vi "test-matrix.vi"(8 "error in (no error)":errorcluster) -> (0 "error out":errorcluster, 3 "All Tests\nPassed":bool)   [LabVIEW 2019]
uses:
  <vilib>/Analysis/baseanly.llb/Real A x B.vi
  <vilib>/Rock Robotics/WPI/ThirdParty/JAS_Junk/TrajLib/MatBuilder_Create.vi
  <vilib>/Analysis/7linalg.llb/Matrix Exp.vi
  <vilib>/Analysis/7linalg.llb/Real Matrix Exp.vi
  <vilib>/Analysis/7linalg.llb/Solve Linear Equations (multiple right hand).vi
  <vilib>/Analysis/baseanly.llb/Real Inverse Matrix.vi
  <vilib>/Analysis/7linalg.llb/Create Special Matrix.vi
  <vilib>/Analysis/7linalg.llb/Create Special Real Matrix.vi
  <vilib>/Analysis/Matrix/Numeric/Add/Add (Elementwise) - RM,R.vi
  <vilib>/Analysis/Matrix/Numeric/Multiply/Multiply - RM,R.vi
  <vilib>/Analysis/Matrix/Numeric/Subtract/Subtract (Elementwise) - RM,R.vi
  <vilib>/Analysis/Matrix/Numeric/Add/Add - RM,RM.vi
  <vilib>/Analysis/Matrix/Numeric/Subtract/Subtract - RM,RM.vi
  <vilib>/Rock Robotics/WPI/ThirdParty/JAS_Junk/TrajLib/Trajectory_Library.lvlib
  <vilib>/Analysis/NI_AALBase.lvlib
  <vilib>/Analysis/NI_AALPro.lvlib
  <vilib>/Analysis/Matrix/NI_Matrix.lvlib
panel:
  out "Test Passed 8-1":bool
  out "Test Passed 8-0":bool
  out "Test Passed 7-1":bool
  out "Test Passed 7-0":bool
  out "Test Passed 6-3":bool
  out "Test Passed 6-2":bool
  out "Test Passed 6-1":bool
  out "Test Passed 6-0":bool
  out "Test Passed 5-0":bool
  out "Test Passed 4-0":bool
  out "Test Passed 3-1":bool
  out "Test Passed 3-0":bool
  out "Test Passed 2-0":bool
  out "Test Passed 1-0":bool
  out "Test Passed 0-1":bool
  out "Test Passed 0-0":bool
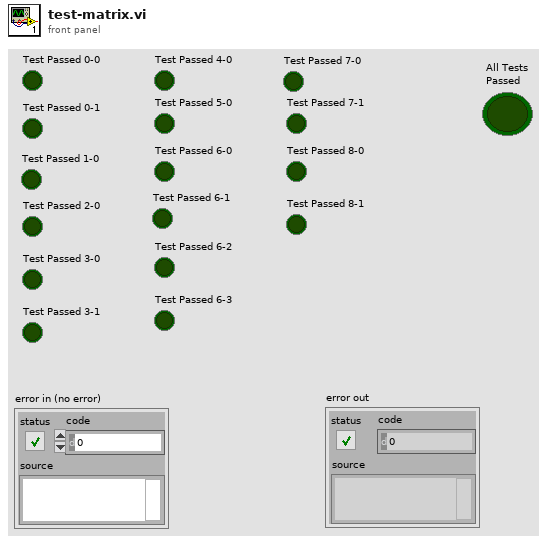
[diagram p1: front panel]
types:
  T1 = typedef "NI_Matrix.lvlib/RealMatrix.ctl" = dbl[][]
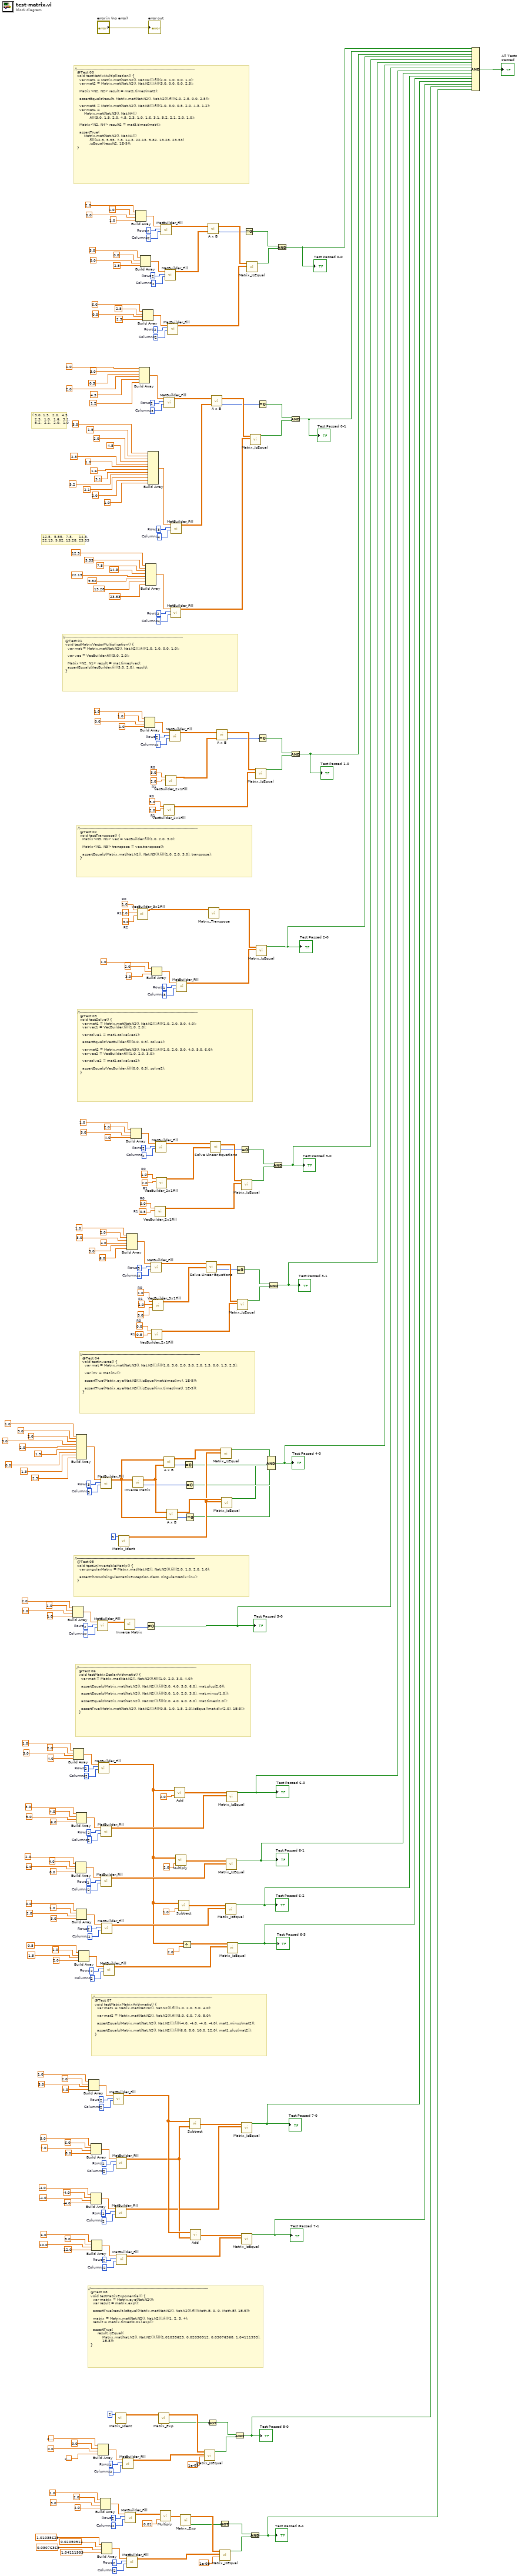
[diagram p0: block diagram]
diagram:
  w13 = 2  # Columns
  w12 = 2  # Rows
  w32 = 2  # Columns
  w31 = 2  # Rows
  w39 = 2  # Columns
  w38 = 2  # Rows
  w50 = 2  # Columns
  w49 = 2  # Rows
  w57 = 2  # Columns
  w56 = 2  # Rows
  w64 = 2  # Columns
  w63 = 2  # Rows
  w71 = 2  # Columns
  w70 = 2  # Rows
  w95 = 2  # Columns
  w94 = 2  # Rows
  w102 = 2  # Columns
  w101 = 2  # Rows
  w109 = 2  # Columns
  w108 = 2  # Rows
  w116 = 2  # Columns
  w115 = 2  # Rows
  w123 = 2  # Columns
  w122 = 2  # Rows
  w133 = 2  # Columns
  w132 = 2  # Rows
  w162 = 3  # Columns
  w161 = 3  # Rows
  w179 = 0.5  # R1
  w178 = 0.0  # R0
  w181 = 2.0  # R1
  w180 = 1.0  # R0
  w183 = 2  # Columns
  w182 = 3  # Rows
  w209 = 0.5  # R1
  w208 = 0.0  # R0
  w211 = 2.0  # R1
  w210 = 1.0  # R0
  w213 = 2  # Columns
  w212 = 2  # Rows
  w225 = 3.0  # R2
  w224 = 2.0  # R1
  w223 = 1.0  # R0
  w227 = 3  # Columns
  w226 = 1  # Rows
  w234 = 2.0  # R1
  w233 = 5.0  # R0
  w237 = 2.0  # R1
  w236 = 3.0  # R0
  w241 = 2  # Columns
  w240 = 2  # Rows
  w265 = 4  # Columns
  w264 = 2  # Rows
  w274 = 4  # Columns
  w273 = 3  # Rows
  w281 = 3  # Columns
  w280 = 2  # Rows
  w290 = 2  # Columns
  w289 = 2  # Rows
  w299 = 2  # Columns
  w298 = 2  # Rows
  w306 = 2  # Columns
  w305 = 2  # Rows
  # "//----------------------------------------------------------------------------------------------------\n  @Test 07\n  void testMatrixMatrixArithmetic() {\n    var mat1 = Matrix.mat(Nat.N2(), Nat.N2()).fill(1.0, 2.0, 3.0, 4.0);\n\n    var mat2 = Matrix.mat(Nat.N2(), Nat.N2()).fill(5.0, 6.0, 7.0, 8.0);\n\n    assertEquals(Matrix.mat(Nat.N2(), Nat.N2()).fill(-4.0, -4.0, -4.0, -4.0), mat1.minus(mat2));\n\n    assertEquals(Matrix.mat(Nat.N2(), Nat.N2()).fill(6.0, 8.0, 10.0, 12.0), mat1.plus(mat2));\n  }"
  # "//----------------------------------------------------------------------------------------------------\n  @Test 06\n  void testMatrixScalarArithmetic() {\n    var mat = Matrix.mat(Nat.N2(), Nat.N2()).fill(1.0, 2.0, 3.0, 4.0);\n\n    assertEquals(Matrix.mat(Nat.N2(), Nat.N2()).fill(3.0, 4.0, 5.0, 6.0), mat.plus(2.0));\n\n    assertEquals(Matrix.mat(Nat.N2(), Nat.N2()).fill(0.0, 1.0, 2.0, 3.0), mat.minus(1.0));\n\n    assertEquals(Matrix.mat(Nat.N2(), Nat.N2()).fill(2.0, 4.0, 6.0, 8.0), mat.times(2.0));\n\n    assertTrue(Matrix.mat(Nat.N2(), Nat.N2()).fill(0.5, 1.0, 1.5, 2.0).isEqual(mat.div(2.0), 1E-3));\n  }"
  # "//----------------------------------------------------------------------------------------------------\n  @Test 05\n  void testUninvertableMatrix() {\n    var singularMatrix = Matrix.mat(Nat.N2(), Nat.N2()).fill(2.0, 1.0, 2.0, 1.0);\n\n    assertThrows(SingularMatrixException.class, singularMatrix::inv);\n  }"
  # "//----------------------------------------------------------------------------------------------------\n  @Test 04\n  void testInverse() {\n    var mat = Matrix.mat(Nat.N3(), Nat.N3()).fill(1.0, 3.0, 2.0, 5.0, 2.0, 1.5, 0.0, 1.3, 2.5);\n\n    var inv = mat.inv();\n\n    assertTrue(Matrix.eye(Nat.N3()).isEqual(mat.times(inv), 1E-9));\n\n    assertTrue(Matrix.eye(Nat.N3()).isEqual(inv.times(mat), 1E-9));\n  }"
  # "//----------------------------------------------------------------------------------------------------\n  @Test 03\n  void testSolve() {\n    var mat1 = Matrix.mat(Nat.N2(), Nat.N2()).fill(1.0, 2.0, 3.0, 4.0);\n    var vec1 = VecBuilder.fill(1.0, 2.0);\n\n    var solve1 = mat1.solve(vec1);\n\n    assertEquals(VecBuilder.fill(0.0, 0.5), solve1);\n\n    var mat2 = Matrix.mat(Nat.N3(), Nat.N2()).fill(1.0, 2.0, 3.0, 4.0, 5.0, 6.0);\n    var vec2 = VecBuilder.fill(1.0, 2.0, 3.0);\n\n    var solve2 = mat2.solve(vec2);\n\n    assertEquals(VecBuilder.fill(0.0, 0.5), solve2);\n  }"
  # "//----------------------------------------------------------------------------------------------------\n  @Test 02\n  void testTranspose() {\n    Matrix<N3, N1> vec = VecBuilder.fill(1.0, 2.0, 3.0);\n\n    Matrix<N1, N3> transpose = vec.transpose();\n\n    assertEquals(Matrix.mat(Nat.N1(), Nat.N3()).fill(1.0, 2.0, 3.0), transpose);\n  }"
  # "//----------------------------------------------------------------------------------------------------\n  @Test 01\n  void testMatrixVectorMultiplication() {\n    var mat = Matrix.mat(Nat.N2(), Nat.N2()).fill(1.0, 1.0, 0.0, 1.0);\n\n    var vec = VecBuilder.fill(3.0, 2.0);\n\n    Matrix<N2, N1> result = mat.times(vec);\n    assertEquals(VecBuilder.fill(5.0, 2.0), result);\n  }"
  # "12.5,  5.55,  7.8,     14.3, \n22.13, 9.82, 13.28, 23.53"
  # "( 3.0, 1.5,  2.0,  4.5, \n  2.3,  1.0,  1.6,  3.1, \n  5.2,  2.1,  2.0,  1.0"
  # "//----------------------------------------------------------------------------------------------------\n  @Test 00\n  void testMatrixMultiplication() {\n    var mat1 = Matrix.mat(Nat.N2(), Nat.N2()).fill(2.0, 1.0, 0.0, 1.0);\n    var mat2 = Matrix.mat(Nat.N2(), Nat.N2()).fill(3.0, 0.0, 0.0, 2.5);\n\n    Matrix<N2, N2> result = mat1.times(mat2);\n\n    assertEquals(result, Matrix.mat(Nat.N2(), Nat.N2()).fill(6.0, 2.5, 0.0, 2.5));\n\n    var mat3 = Matrix.mat(Nat.N2(), Nat.N3()).fill(1.0, 3.0, 0.5, 2.0, 4.3, 1.2);\n    var mat4 =\n        Matrix.mat(Nat.N3(), Nat.N4())\n            .fill(3.0, 1.5, 2.0, 4.5, 2.3, 1.0, 1.6, 3.1, 5.2, 2.1, 2.0, 1.0);\n\n    Matrix<N2, N4> result2 = mat3.times(mat4);\n\n    assertTrue(\n        Matrix.mat(Nat.N2(), Nat.N4())\n            .fill(12.5, 5.55, 7.8, 14.3, 22.13, 9.82, 13.28, 23.53)\n            .isEqual(result2, 1E-9));\n  }"
  # "//----------------------------------------------------------------------------------------------------\n  @Test 08\n  void testMatrixExponential() {\n    var matrix = Matrix.eye(Nat.N2());\n    var result = matrix.exp();\n\n    assertTrue(result.isEqual(Matrix.mat(Nat.N2(), Nat.N2()).fill(Math.E, 0, 0, Math.E), 1E-9));\n\n    matrix = Matrix.mat(Nat.N2(), Nat.N2()).fill(1, 2, 3, 4);\n    result = matrix.times(0.01).exp();\n\n    assertTrue(\n        result.isEqual(\n            Matrix.mat(Nat.N2(), Nat.N2()).fill(1.01035625, 0.02050912, 0.03076368, 1.04111993),\n            1E-8));\n  }"
  n1 = Build Array(2.0 ("element"), 1.0 ("element"), 2.0 ("element"), 1.0 ("element")) -> (w138:dbl[])
  n2 = Build Array(1.0 ("element"), 2.0 ("element"), 3.0 ("element"), 4.0 ("element")) -> (w128:dbl[])
  n3 = Build Array(2.0 ("element"), 4.0 ("element"), 6.0 ("element"), 8.0 ("element")) -> (w114:dbl[])
  n4 = Build Array(1.0 ("element"), 3.0 ("element"), 2.0 ("element"), 5.0 ("element"), 2.0 ("element"), 1.5 ("element"), 0.0 ("element"), 1.3 ("element"), 2.5 ("element")) -> (w167:dbl[])
  n5 = Build Array(3.0 ("element"), 4.0 ("element"), 5.0 ("element"), 6.0 ("element")) -> (w121:dbl[])
  n6 = Build Array(0.0 ("element"), 1.0 ("element"), 2.0 ("element"), 3.0 ("element")) -> (w107:dbl[])
  n7 = Build Array(0.5 ("element"), 1.0 ("element"), 1.5 ("element"), 2.0 ("element")) -> (w100:dbl[])
  n8 = Build Array(1.0 ("element"), 2.0 ("element"), 3.0 ("element"), 4.0 ("element")) -> (w76:dbl[])
  n9 = Build Array(-4.0 ("element"), -4.0 ("element"), -4.0 ("element"), -4.0 ("element")) -> (w62:dbl[])
  n10 = Build Array(5.0 ("element"), 6.0 ("element"), 7.0 ("element"), 8.0 ("element")) -> (w69:dbl[])
  n11 = Build Array(6.0 ("element"), 8.0 ("element"), 10.0 ("element"), 12.0 ("element")) -> (w55:dbl[])
  n12 = call <vilib>:"MatBuilder_Fill.vi"("Columns"=w133, "Rows"=w132, "Value List"=w138) -> ("output matrix"=w131:T1)  [unwired: 8 in]
  n13 = Build Array(2.718281828459045, 0.0 ("element"), 0.0 ("element"), 2.718281828459045) -> (w42:dbl[])
  n14 = call <vilib>:"MatBuilder_Fill.vi"("Columns"=w123, "Rows"=w122, "Value List"=w128) -> ("output matrix"=w83:T1)  [unwired: 8 in]
  n15 = Build Array(1.0 ("element"), 2.0 ("element"), 3.0 ("element"), 4.0 ("element")) -> (w37:dbl[])
  n16 = call <vilib>:"MatBuilder_Fill.vi"("Columns"=w109, "Rows"=w108, "Value List"=w114) -> ("output matrix"=w88:T1)  [unwired: 8 in]
  n17 = call <vilib>:"MatBuilder_Fill.vi"("Columns"=w162, "Rows"=w161, "Value List"=w167) -> ("output matrix"=w154:T1)  [unwired: 8 in]
  n18 = call <vilib>:"MatBuilder_Fill.vi"("Columns"=w116, "Rows"=w115, "Value List"=w121) -> ("output matrix"=w91:T1)  [unwired: 8 in]
  n19 = call <vilib>:"MatBuilder_Fill.vi"("Columns"=w102, "Rows"=w101, "Value List"=w107) -> ("output matrix"=w85:T1)  [unwired: 8 in]
  n20 = Build Array(1.01035625 ("element"), 0.02050912 ("element"), 0.03076368 ("element"), 1.04111993 ("element")) -> (w18:dbl[])
  n21 = call <vilib>:"MatBuilder_Fill.vi"("Columns"=w95, "Rows"=w94, "Value List"=w100) -> ("output matrix"=w81:T1)  [unwired: 8 in]
  n22 = call <vilib>:"MatBuilder_Fill.vi"("Columns"=w71, "Rows"=w70, "Value List"=w76) -> ("output matrix"=w46:T1)  [unwired: 8 in]
  n23 = call <vilib>:"Matrix_Ident.vi"("Size"=2) -> ("output matrix"=w28:T1)  [unwired: 9 in, 1 out]
  n24 = call <vilib>:"MatBuilder_Fill.vi"("Columns"=w57, "Rows"=w56, "Value List"=w62) -> ("output matrix"=w44:T1)  [unwired: 8 in]
  n25 = call <vilib>:"MatBuilder_Fill.vi"("Columns"=w64, "Rows"=w63, "Value List"=w69) -> ("output matrix"=w45:T1)  [unwired: 8 in]
  n26 = call <vilib>:"MatBuilder_Fill.vi"("Columns"=w50, "Rows"=w49, "Value List"=w55) -> ("output matrix"=w43:T1)  [unwired: 8 in]
  n27 = call <vilib>:"Matrix_Ident.vi"("Size"=3) -> ("output matrix"=w147:T1)  [unwired: 9 in, 1 out]
  n28 = call <vilib>:"MatBuilder_Fill.vi"("Columns"=w39, "Rows"=w38, "Value List"=w42) -> ("output matrix"=w24:T1)  [unwired: 8 in]
  n29 = call-poly <vilib>:"Inverse Matrix.vi"("Input Matrix"=w131) -> ("error"=w130:i32)  [unwired: 1 in, 1 out]
  n30 = call <vilib>:"MatBuilder_Fill.vi"("Columns"=w32, "Rows"=w31, "Value List"=w37) -> ("output matrix"=w22:T1)  [unwired: 8 in]
  n31 = Build Array(1.0 ("element"), 2.0 ("element"), 3.0 ("element"), 4.0 ("element"), 5.0 ("element"), 6.0 ("element")) -> (w188:dbl[])
  n32 = call <vilib>:"MatBuilder_Fill.vi"("Columns"=w13, "Rows"=w12, "Value List"=w18) -> ("output matrix"=w11:T1)  [unwired: 8 in]
  n33 = Build Array(1.0 ("element"), 2.0 ("element"), 3.0 ("element"), 4.0 ("element")) -> (w218:dbl[])
  n34 = call-poly <vilib>:"Inverse Matrix.vi"("Input Matrix"=w154) -> ("error"=w152:i32, "Inverse Matrix"=w155:T1)  [unwired: 1 in]
  n35 = Build Array(2.0 ("element"), 1.0 ("element"), 0.0 ("element"), 1.0 ("element")) -> (w311:dbl[])
  n36 = call <vilib>:"VecBuilder_3x1Fill.vi"("R2"=w225, "R1"=w224, "R0"=w223) -> ("output matrix"=w221:T1)  [unwired: 8 in]
  n37 = Build Array(1.0 ("element"), 3.0 ("element"), 0.5 ("element"), 2.0 ("element"), 4.3 ("element"), 1.2 ("element")) -> (w286:dbl[])
  n38 = Build Array(3.0 ("element"), 0.0 ("element"), 0.0 ("element"), 2.5 ("element")) -> (w304:dbl[])
  n39 = Build Array(6.0 ("element"), 2.5 ("element"), 0.0 ("element"), 2.5 ("element")) -> (w295:dbl[])
  n40 = Build Array(1.0 ("element"), 1.0 ("element"), 0.0 ("element"), 1.0 ("element")) -> (w246:dbl[])
  n41 = Build Array(12.5 ("element"), 5.55 ("element"), 7.8 ("element"), 14.3 ("element"), 22.13 ("element"), 9.82 ("element"), 13.28 ("element"), 23.53 ("element")) -> (w270:dbl[])
  n42 = Not Equal To 0?(x=w130) -> (x != 0?=w129:bool)
  "Test Passed 5-0" <- w129
  n43 = Build Array(3.0 ("element"), 1.5 ("element"), 2.0 ("element"), 4.5 ("element"), 2.3 ("element"), 1.0 ("element"), 1.6 ("element"), 3.1 ("element"), 5.2 ("element"), 2.1 ("element"), 2.0 ("element"), 1.0 ("element")) -> (w279:dbl[])
  n44 = call <vilib>:"MatBuilder_Fill.vi"("Columns"=w183, "Rows"=w182, "Value List"=w188) -> ("output matrix"=w176:T1)  [unwired: 8 in]
  n45 = Build Array(1.0 ("element"), 2.0 ("element"), 3.0 ("element")) -> (w231:dbl[])
  n46 = call <vilib>:"VecBuilder_2x1Fill.vi"("R1"=w179, "R0"=w178) -> ("output matrix"=w177:T1)  [unwired: 9 in]
  n47 = call <vilib>:"VecBuilder_3x1Fill.vi"("R2"=3.0, "R1"=w181, "R0"=w180) -> ("output matrix"=w175:T1)  [unwired: 8 in]
  n48 = call <vilib>:"VecBuilder_2x1Fill.vi"("R1"=w209, "R0"=w208) -> ("output matrix"=w207:T1)  [unwired: 9 in]
  n49 = call <vilib>:"MatBuilder_Fill.vi"("Columns"=w213, "Rows"=w212, "Value List"=w218) -> ("output matrix"=w206:T1)  [unwired: 8 in]
  n50 = call <vilib>:"VecBuilder_2x1Fill.vi"("R1"=w211, "R0"=w210) -> ("output matrix"=w205:T1)  [unwired: 9 in]
  n51 = call <vilib>:"Matrix_Exp.vi"("input matrix"=w28) -> ("Error"=w4:bool, "output matrix"=w27:T1)  [unwired: 9 in]
  n52 = call-poly <vilib>:"Multiply.vi"("Real Scalar c"=0.01 ("y"), "Real Matrix A"=w22) -> ("A * c"=w19:T1)
  n53 = call <vilib>:"MatBuilder_Fill.vi"("Columns"=w306, "Rows"=w305, "Value List"=w311) -> ("output matrix"=w297:T1)  [unwired: 8 in]
  n54 = call-poly <vilib>:"A x B.vi"("B"=w155, "A"=w154) -> ("error"=w151:i32, "A x B"=w148:T1)
  n55 = call <vilib>:"MatBuilder_Fill.vi"("Columns"=w281, "Rows"=w280, "Value List"=w286) -> ("output matrix"=w272:T1)  [unwired: 8 in]
  n56 = call <vilib>:"VecBuilder_2x1Fill.vi"("R1"=w234, "R0"=w233) -> ("output matrix"=w232:T1)  [unwired: 9 in]
  n57 = call <vilib>:"MatBuilder_Fill.vi"("Columns"=w299, "Rows"=w298, "Value List"=w304) -> ("output matrix"=w296:T1)  [unwired: 8 in]
  n58 = call <vilib>:"VecBuilder_2x1Fill.vi"("R1"=w237, "R0"=w236) -> ("output matrix"=w235:T1)  [unwired: 9 in]
  n59 = call-poly <vilib>:"A x B.vi"("B"=w154, "A"=w155) -> ("error"=w150:i32, "A x B"=w149:T1)
  n60 = call <vilib>:"MatBuilder_Fill.vi"("Columns"=w290, "Rows"=w289, "Value List"=w295) -> ("output matrix"=w287:T1)  [unwired: 8 in]
  n61 = call <vilib>:"MatBuilder_Fill.vi"("Columns"=w241, "Rows"=w240, "Value List"=w246) -> ("output matrix"=w239:T1)  [unwired: 8 in]
  n62 = call <vilib>:"MatBuilder_Fill.vi"("Columns"=w265, "Rows"=w264, "Value List"=w270) -> ("output matrix"=w262:T1)  [unwired: 8 in]
  n63 = call <vilib>:"MatBuilder_Fill.vi"("Columns"=w274, "Rows"=w273, "Value List"=w279) -> ("output matrix"=w271:T1)  [unwired: 8 in]
  n64 = call-poly <vilib>:"Add.vi"("Real Scalar c"=2.0 ("y"), "Real Matrix A"=w83) -> ("A + c"=w92:T1)
  n65 = call-poly <vilib>:"Multiply.vi"("Real Scalar c"=2.0 ("y"), "Real Matrix A"=w83) -> ("A * c"=w89:T1)
  n66 = call <vilib>:"MatBuilder_Fill.vi"("Columns"=w227, "Rows"=w226, "Value List"=w231) -> ("output matrix"=w220:T1)  [unwired: 8 in]
  n67 = call-poly <vilib>:"Subtract.vi"("Real Scalar c"=1.0 ("y"), "Real Matrix A"=w83) -> ("A - c"=w86:T1)
  n68 = call <vilib>:"Matrix_Exp.vi"("input matrix"=w19) -> ("Error"=w2:bool, "output matrix"=w20:T1)  [unwired: 9 in]
  n69 = Divide(x=w83, y=2.0) -> (x/y=w82:T1)
  n70 = Equal To 0?(x=w151) -> (x = 0?=w145:bool)
  n71 = Equal To 0?(x=w152) -> (x = 0?=w144:bool)
  n72 = Equal To 0?(x=w150) -> (x = 0?=w142:bool)
  n73 = call-poly <vilib>:"Subtract.vi"("Real Matrix B"=w45, "Real Matrix A"=w46) -> ("A - B"=w48:T1)
  n74 = call-poly <vilib>:"Add.vi"("Real Matrix B"=w45, "Real Matrix A"=w46) -> ("A + B"=w47:T1)
  n75 = call <vilib>:"Matrix_IsEqual.vi"("Tolerance"=1e-09, "other"=w24, "input matrix"=w27) -> ("Equal"=w30:bool)  [unwired: 8 in]
  n76 = call-poly <vilib>:"Solve Linear Equations.vi"("Known Matrix"=w175, "Input Matrix"=w176) -> ("error"=w173:i32, "Solution Matrix"=w174:T1)  [unwired: 1 in]
  n77 = Not(x=w4) -> (.not. x?=w3:bool)
  n78 = call-poly <vilib>:"A x B.vi"("B"=w296, "A"=w297) -> ("error"=w191:i32, "A x B"=w288:T1)
  n79 = call <vilib>:"Matrix_Transpose.vi"("input matrix"=w221) -> ("output matrix"=w222:T1)  [unwired: 10 in]
  n80 = call-poly <vilib>:"Solve Linear Equations.vi"("Known Matrix"=w205, "Input Matrix"=w206) -> ("error"=w203:i32, "Solution Matrix"=w204:T1)  [unwired: 1 in]
  n81 = call-poly <vilib>:"A x B.vi"("B"=w271, "A"=w272) -> ("error"=w195:i32, "A x B"=w263:T1)
  n82 = call-poly <vilib>:"A x B.vi"("B"=w235, "A"=w239) -> ("error"=w199:i32, "A x B"=w238:T1)
  n83 = Not(x=w2) -> (.not. x?=w1:bool)
  n84 = call <vilib>:"Matrix_IsEqual.vi"("Tolerance"=1e-08, "other"=w11, "input matrix"=w20) -> ("Equal"=w21:bool)  [unwired: 8 in]
  n85 = call <vilib>:"Matrix_IsEqual.vi"("other"=w147, "input matrix"=w148) -> ("Equal"=w146:bool)  [unwired: 9 in]
  n86 = call <vilib>:"Matrix_IsEqual.vi"("other"=w147, "input matrix"=w149) -> ("Equal"=w143:bool)  [unwired: 9 in]
  n87 = call <vilib>:"Matrix_IsEqual.vi"("other"=w85, "input matrix"=w86) -> ("Equal"=w78:bool)  [unwired: 9 in]
  "Test Passed 6-2" <- w78
  n88 = call <vilib>:"Matrix_IsEqual.vi"("other"=w88, "input matrix"=w89) -> ("Equal"=w79:bool)  [unwired: 9 in]
  "Test Passed 6-1" <- w79
  n89 = call <vilib>:"Matrix_IsEqual.vi"("other"=w91, "input matrix"=w92) -> ("Equal"=w80:bool)  [unwired: 9 in]
  "Test Passed 6-0" <- w80
  n90 = call <vilib>:"Matrix_IsEqual.vi"("other"=w81, "input matrix"=w82) -> ("Equal"=w77:bool)  [unwired: 9 in]
  "Test Passed 6-3" <- w77
  n91 = And(x=w3, y=w30) -> (x .and. y?=w6:bool)
  "Test Passed 8-0" <- w6
  n92 = Equal To 0?(x=w173) -> (x = 0?=w171:bool)
  n93 = call <vilib>:"Matrix_IsEqual.vi"("other"=w177, "input matrix"=w174) -> ("Equal"=w172:bool)  [unwired: 9 in]
  n94 = Equal To 0?(x=w203) -> (x = 0?=w201:bool)
  n95 = call <vilib>:"Matrix_IsEqual.vi"("other"=w43, "input matrix"=w47) -> ("Equal"=w7:bool)  [unwired: 9 in]
  "Test Passed 7-1" <- w7
  n96 = call <vilib>:"Matrix_IsEqual.vi"("other"=w207, "input matrix"=w204) -> ("Equal"=w202:bool)  [unwired: 9 in]
  n97 = call <vilib>:"Matrix_IsEqual.vi"("other"=w44, "input matrix"=w48) -> ("Equal"=w8:bool)  [unwired: 9 in]
  "Test Passed 7-0" <- w8
  n98 = Equal To 0?(x=w191) -> (x = 0?=w192:bool)
  n99 = call <vilib>:"Matrix_IsEqual.vi"("other"=w287, "input matrix"=w288) -> ("Equal"=w190:bool)  [unwired: 9 in]
  n100 = call <vilib>:"Matrix_IsEqual.vi"("other"=w262, "input matrix"=w263) -> ("Equal"=w194:bool)  [unwired: 9 in]
  n101 = And(x=w1, y=w21) -> (x .and. y?=w5:bool)
  "Test Passed 8-1" <- w5
  n102 = call <vilib>:"Matrix_IsEqual.vi"("other"=w232, "input matrix"=w238) -> ("Equal"=w197:bool)  [unwired: 9 in]
  n103 = call <vilib>:"Matrix_IsEqual.vi"("other"=w220, "input matrix"=w222) -> ("Equal"=w219:bool)  [unwired: 9 in]
  "Test Passed 2-0" <- w219
  n104 = Equal To 0?(x=w195) -> (x = 0?=w196:bool)
  n105 = Equal To 0?(x=w199) -> (x = 0?=w200:bool)
  n106 = Compound Arithmetic op=AND(w146, w145, w144, w143, w142) -> (w139:bool)
  "Test Passed 4-0" <- w139
  n107 = And(x=w171, y=w172) -> (x .and. y?=w140:bool)
  "Test Passed 3-1" <- w140
  n108 = And(x=w201, y=w202) -> (x .and. y?=w141:bool)
  "Test Passed 3-0" <- w141
  n109 = And(x=w192, y=w190) -> (x .and. y?=w189:bool)
  "Test Passed 0-0" <- w189
  n110 = And(x=w196, y=w194) -> (x .and. y?=w193:bool)
  "Test Passed 0-1" <- w193
  n111 = And(x=w200, y=w197) -> (x .and. y?=w198:bool)
  "Test Passed 1-0" <- w198
  n112 = Compound Arithmetic op=AND(w189, w193, w198, w219, w141, w140, w139, w129, w80, w79, w78, w77, w8, w7, w6, w5) -> (→"All Tests\nPassed":bool)
  "error out" <- "error in (no error)"
